vi "Waveform_Resample with new dt.vi"(10 "new dt":dbl, 11 "Waveform to Merge in":T1) -> (3 "Waveform to Merge out":T1)   [LabVIEW 2020]
uses:
  Universal Controls/Waveform_Data.ctl
  <vilib>/Waveform/WDTOps.llb/WDT Waveform Duration DBL.vi
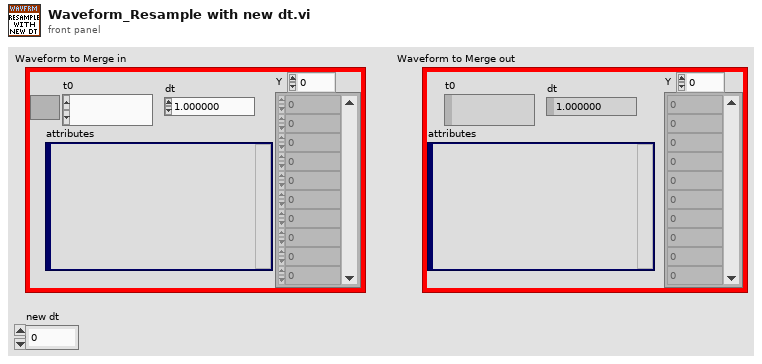
[diagram p1: front panel]
types:
  T1 = typedef "Waveform_Data.ctl" = waveform(dbl)
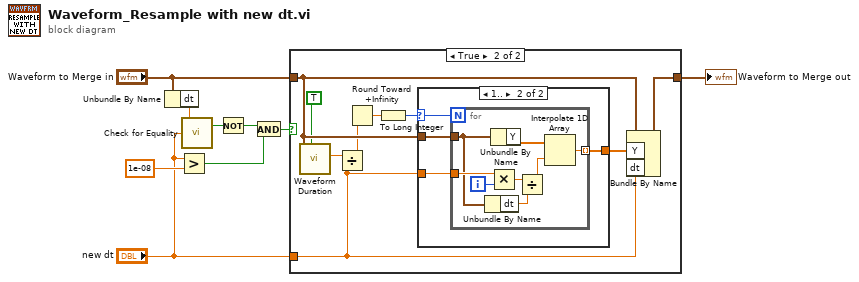
[diagram p0: block diagram]
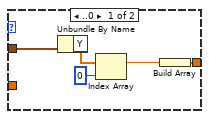
[diagram p3: hidden frame]
diagram:
  n1 = Unbundle By Name("Waveform to Merge in") -> ("dt"=w4:dbl)
  n2 = Greater?(x="new dt", y=1e-08) -> (0:w5:bool)
  n3 = call <vilib>:"Check for Equality.vi"("n2"="new dt", "n1"=w4) -> ("equal?"=w3:bool)  [unwired: 1 in, 1 out]
  n4 = Not(x=w3) -> (.not. x?=w2:bool)
  n5 = And(x=w2, y=w5) -> (x .and. y?=w6:bool)
  n6 = case shown="True" w6 {
    tunnel: [w10 w19] -> w8
    tunnel: "Waveform to Merge in" -> [w10 w17]
    tunnel: "new dt" -> [_ w18]
    frame False {
    }
    frame True {
      n7 = call-poly <vilib>:"Waveform Duration.vi"("open interval? (T)"=TRUE, "waveform in"=w17) -> ("duration"=w16:dbl)  [unwired: 7 in, 2 out]
      n8 = Divide(x=w16, y=w18) -> (x/y=w15:dbl)
      n9 = Round Toward +Infinity(x=w15) -> (ceil(x): smallest int >= x=w14:dbl)
      n10 = To Long Integer(number=w14) -> (32bit integer=w11:i32)
      n11 = case shown="1.." w11 {
        selector: w11 -> [_ w25]
        tunnel: w18 -> [_ w28]
        tunnel: w17 -> [w24 w27]
        tunnel: [w20 w26] -> w13
        frame ..0 {
          n12 = Unbundle By Name(w24) -> ("Y"=w23:dbl[])
          n13 = Index Array(array=w23, index=0) -> (element=w21:dbl)
          n14 = Build Array(w21) -> (w20:dbl[])
        }
        frame 1.. {
          n15 = for {
            N: w25 -> [_]
            tunnel: w27 -> [w34]
            tunnel: w28 -> [w35]
            tunnel: [w30] -> w26 mode=indexing
            i -> [w33]
            n16 = Unbundle By Name(w34) -> ("dt"=w31:dbl)
            n17 = Multiply(x=w35, y=w33) -> (x*y=w32:dbl)
            n18 = Unbundle By Name(w34) -> ("Y"=w36:dbl[])
            n19 = Divide(x=w32, y=w31) -> (x/y=w29:dbl)
            n20 = Interpolate 1D Array(1:w29, 2:w36) -> (0:w30:dbl)
          }
        }
      }
      n21 = Bundle By Name(cluster=w17, "Y"=w13, "dt"=w18) -> (w19:T1)
    }
  }
  "Waveform to Merge out" <- w8
